vi "FRCts20_Backend_Dyn_Launcher.vi"(6 "Message Attributes":T4, 7 "VI Name":path, 8 "error in (no error)":errorcluster, 10 "Data":string, 11 "Engine_Refnums":T1) -> (0 "error out":errorcluster)   [LabVIEW 2013, in "FRCts20_Backend_Engine.lvlib"]
uses:
  FRCts20_Backend_Engine.lvlib
  Dependencies/Keyed Array/KeyedArray.ctl
  FRCts20_Backend_EngineRefnums.ctl
  INI_Accessor/FRCts20_Backend_INI Controller.lvclass
  Dependencies/AMC/_SubVIs/TypeDefs/Message Queue.ctl
  Dependencies/AMC/_SubVIs/TypeDefs/Message.ctl
  <vilib>/addons/database/Connection.llb/Conn ObjectReference.ctl
  FRCts20_Backend_Dyn_FGV_Command.ctl
  FRCts20_Backend_Dyn_Refnums.ctl
  Dependencies/Keyed Array/Tools_KeyedArray.lvlib
  Dependencies/AMC/AMC.lvlib
  <vilib>/addons/database/NI_Database_API.lvlib
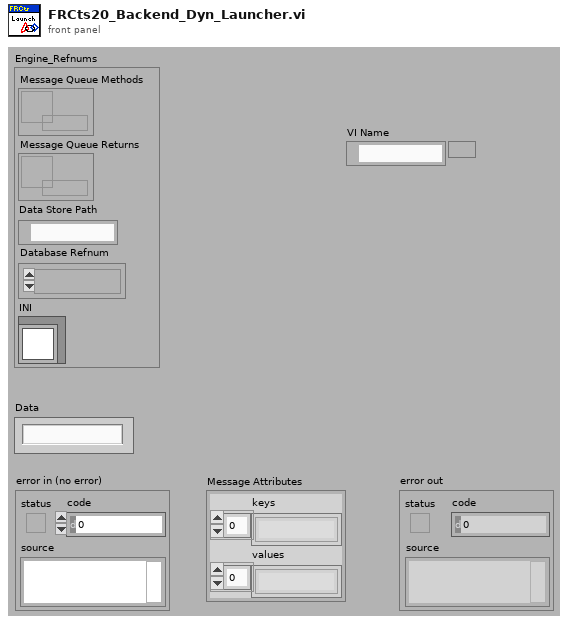
[diagram p1: front panel]
types:
  T1 = typedef "FRCts20_Backend_Engine.lvlib/FRCts20_Backend_EngineRefnums.ctl" = cluster{"Message Queue Methods":T2, "Message Queue Returns":T2, "Data Store Path":path, "Database Refnum":T3, "INI":refnum<class "FRCts20_Backend_INI Controller.lvclass">}
  T2 = typedef "AMC.lvlib/Message Queue.ctl" = refnum<queue>
  T3 = typedef "NI_Database_API.lvlib/Conn ObjectReference.ctl" = refnum<k1>
  T4 = typedef "Tools_KeyedArray.lvlib/KeyedArray.ctl" = cluster{"keys":string[], "values":string[]}
  T5 = typedef "FRCts20_Backend_Engine.lvlib/FRCts20_Backend_Dyn_FGV_Command.ctl" = enum16{"Load", "Locate", "Unload"}
  T6 = typedef "FRCts20_Backend_Engine.lvlib/FRCts20_Backend_Dyn_Refnums.ctl" = cluster{"VI Name":path, "vi reference":refnum<vi>}
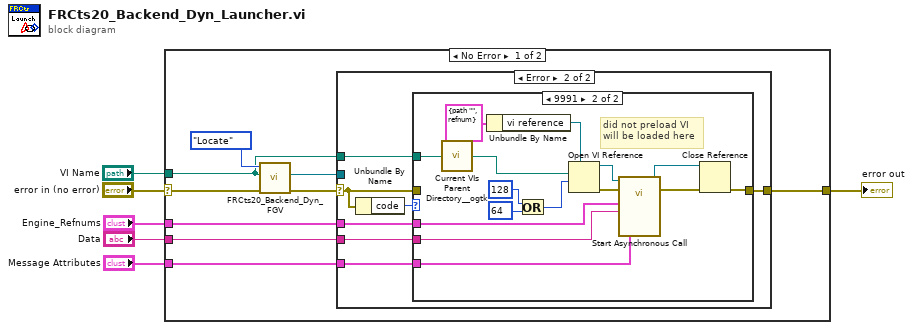
[diagram p0: block diagram]
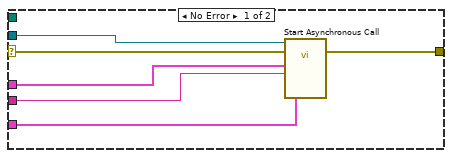
[diagram p2: hidden frame]
diagram:
  n1 = case shown="No Error" "error in (no error)" {
    selector: "error in (no error)" -> [w14 w45]
    tunnel: [w15 w45] -> w5
    tunnel: "VI Name" -> [w7 _]
    tunnel: "Engine_Refnums" -> [w10 _]
    tunnel: "Data" -> [w9 _]
    tunnel: "Message Attributes" -> [w8 _]
    frame No Error {
      n2 = call "FRCts20_Backend_Dyn_FGV.vi"("error in"=w14, "VI to Locate"=w7, "Command"=FRCts20_Backend_Dyn_FGV_Command."Locate") -> ("error out"=w11:errorcluster, "vi reference"=w12:refnum<vi>)  [unwired: 6 in, 1 out]
      n3 = case shown="Error" w11 {
        selector: w11 -> [w19 w27]
        tunnel: [w21 w26] -> w15
        tunnel: w12 -> [w20 _]
        tunnel: w10 -> [w18 w23]
        tunnel: w9 -> [w17 w22]
        tunnel: w8 -> [w16 w24]
        tunnel: w7 -> [_ w25]
        frame No Error {
          n4 = call-by-ref "Start Asynchronous Call"(reference=w20, error in=w19, "Message Attributes"=w16, "Data"=w17, "Engine_Refnums"=w18) -> (error out=w21:errorcluster)  [unwired: 8 in, 2 out]
        }
        frame Error {
          n5 = Unbundle By Name(w27) -> ("code"=w28:i32)
          n6 = case shown="9991" w28 {
            tunnel: w27 -> [w29 _]
            tunnel: [w29 w34] -> w26
            tunnel: w25 -> [_ w30]
            tunnel: w24 -> [_ w33]
            tunnel: w23 -> [_ w32]
            tunnel: w22 -> [_ w31]
            frame 0, Default {
              # "error code is not the error\nfrom being unable to find\nthe vi in question"
            }
            frame 9991 {
              # "did not preload VI\nwill be loaded here"
              n7 = call "Current VIs Parent Directory__ogtk.vi"("Relative path (.)"=w30) -> ("Parent Directory (+ Relative)"=w44:path)  [unwired: 4 in]
              n8 = Unbundle By Name(T6 {"VI Name"=path "", "vi reference"=refnum} ("Dynamic VIs")) -> ("vi reference"=w42:refnum<vi>)
              n9 = Or(x=128, y=64) -> (x .or. y?=w39:i32)
              n10 = Open VI Reference(type specifier VI Refnum (for type only)=w42, vi path=w44, options=w39) -> (vi reference=w38:refnum<vi>, error out=w37:errorcluster)  [unwired: 3 in]
              n11 = call-by-ref "Start Asynchronous Call"(reference=w38, error in=w37, "Message Attributes"=w33, "Data"=w31, "Engine_Refnums"=w32) -> (reference out=w36:refnum<vi>, error out=w35:errorcluster)  [unwired: 8 in, 1 out]
              n12 = Close Reference(reference=w36, error in (no error)=w35) -> (error out=w34:errorcluster)
            }
          }
        }
      }
    }
    frame Error {
    }
  }
  "error out" <- w5
